vi "Set Port Status.vi"(8 "error in (no error)":errorcluster, 9 "Value":string, 10 "Port":dbl, 11 "NXP in":refnum<class "NXP.lvclass">) -> (0 "error out":errorcluster, 3 "NXP out":refnum<class "NXP.lvclass">)   [LabVIEW 2020, in "NXP.lvclass"]
doc: "Método heredado del padre con un override"
uses:
  NXP.lvclass
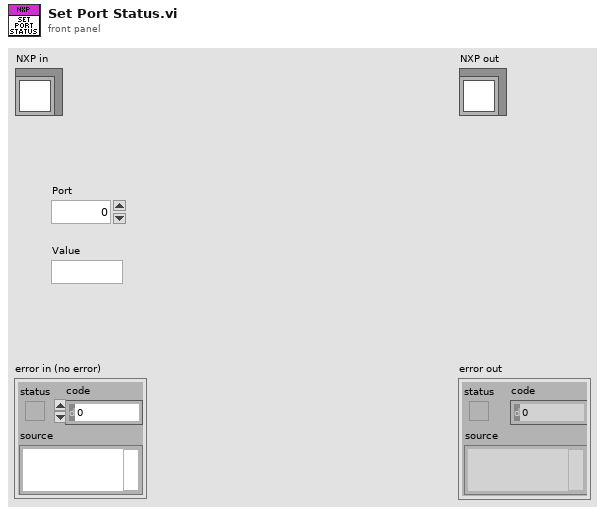
[diagram p1: front panel]
types:
  T1 = typedef "Serial device.lvclass/Brand combobox.ctl" = string
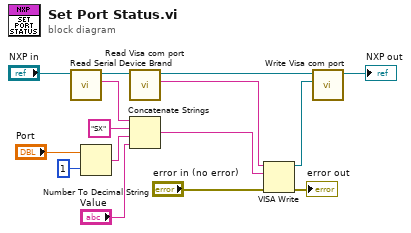
[diagram p0: block diagram]
diagram:
  n1 = call-dynamic "Read Serial Device Brand.vi"("Serial device in"="NXP in") -> ("Serial Device Brand"=w13:T1, "Serial device out"=w15:refnum<class "NXP.lvclass">)  [unwired: 8 in, 1 out]
  n2 = Number To Decimal String(number="Port", width (-)=i16 1) -> (decimal integer string=w9:string)
  n3 = call-dynamic "Read Visa com port.vi"("Serial device in"=w15) -> ("Visa com port"=w6:string, "Serial device out"=w5:refnum<class "NXP.lvclass">)  [unwired: 8 in, 1 out]
  n4 = Concatenate Strings(w13, "SX" ("string"), w9, "Value") -> (w7:string)
  n5 = VISA Write(VISA resource name=w6, write buffer=w7, error in (no error)="error in (no error)") -> (VISA resource name out=w4:refnum<visa-resource-name>, error out=→"error out":errorcluster)  [unwired: 1 out]
  n6 = call-dynamic "Write Visa com port.vi"("Visa com port"=w4, "Serial device in"=w5) -> ("Serial device out"=→"NXP out":refnum<class "NXP.lvclass">)  [unwired: 8 in, 1 out]
